vi "FGV Modbus_F.vi"(6 "Aktion":T1) -> (0 "error out":errorcluster)   [LabVIEW 2020, in "ABB-EL3000.lvlib" / "FID.lvlib"]
uses:
  FID.lvlib
  Aktion FGV Modbus_F.ctl
  Aktion Adressen_F.ctl
  Aktion STY_MES.ctl
  Aktion FGV Messwerte_F.ctl
  Allgemeine VI/Aktion Modbus lesen.ctl
  Status Analysatoren/Aktion Status Analysatoren.ctl
  FID Kalibrierung/Aktion FID Allgemeindaten.ctl
  Allgemeine VI/Allgemeine VI.lvlib
  FID Kalibrierung/FID Kalibrierung.lvlib
  Status Analysatoren/Status Analysatoren.lvlib
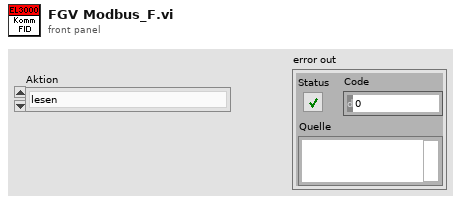
[diagram p1: front panel]
types:
  T1 = typedef "ABB-EL3000.lvlib/FID.lvlib/Aktion FGV Modbus_F.ctl" = enum16{"lesen", "Verbindung herstellen", "Verbindung trennen", "Komm"}
  T2 = typedef "ABB-EL3000.lvlib/FID.lvlib/Aktion Adressen_F.ctl" = enum16{"lesen", "initialisieren"}
  T3 = typedef "Status Analysatoren.lvlib/Aktion Status Analysatoren.ctl" = enum16{"lesen", "initialisieren", "Analysatoren aktiv", "FTIR Fehler", "FID Fehler", "PMA Fehler", "Felder einfärben"}
  T4 = typedef "ABB-EL3000.lvlib/Allgemeine VI.lvlib/Aktion Modbus lesen.ctl" = enum16{"Coils", "Discrete Inputs", "Input Register", "Holding Register"}
  T5 = typedef "ABB-EL3000.lvlib/FID.lvlib/Aktion FGV Messwerte_F.ctl" = enum16{"lesen", "Messwerte", "Messbereich", "Status", "Diagnose Werte"}
  T6 = typedef "Aktion STY_MES.ctl" = enum16{"lesen", "setze STY", "setze MES", "MODBUS schreiben"}
  T7 = typedef "ABB-EL3000.lvlib/FID.lvlib/FID Kalibrierung.lvlib/Aktion FID Allgemeindaten.ctl" = enum16{"lesen", "Mod", "Time", "laden", "speichern"}
  T8 = typedef "Status Analysatoren.lvlib/Status.ctl" = cluster{"FT-IR aktiv":bool, "FT-IR Fehler":bool, "FID aktiv":bool, "FID Fehler":bool, "PMA aktiv":bool, "PMA Fehler":bool}
  T9 = typedef "ABB-EL3000.lvlib/FID.lvlib/Modus.ctl" = enum16{"Automatic", "CH4", "THC", "Efficienty measure", "Switching time"}
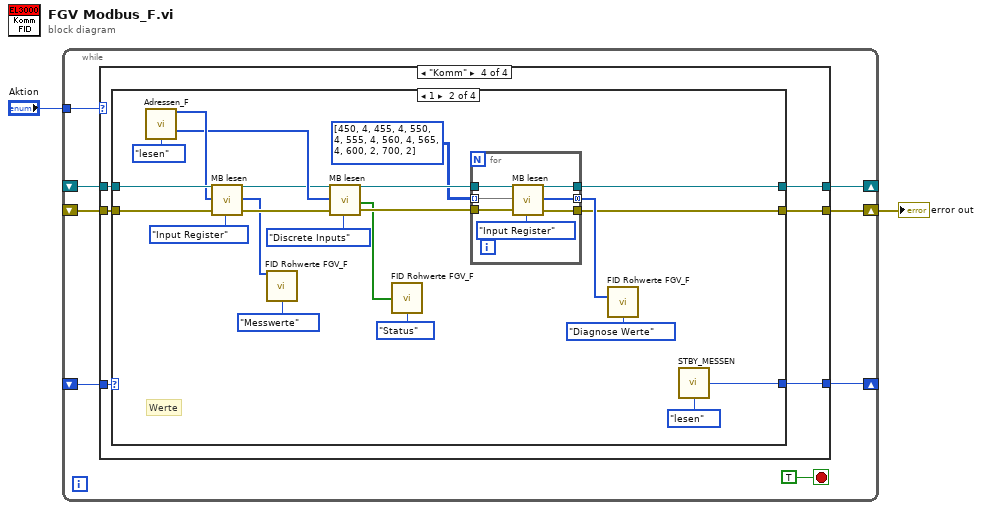
[diagram p0: block diagram]
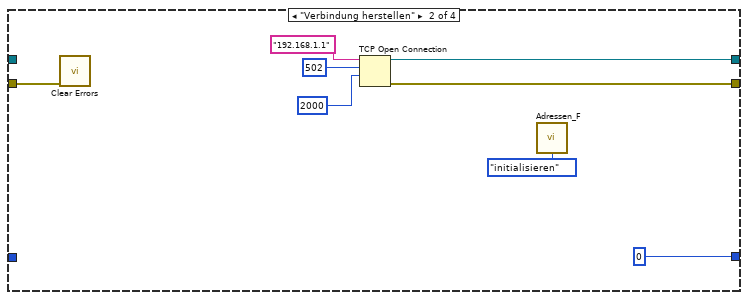
[diagram p3: hidden frame]
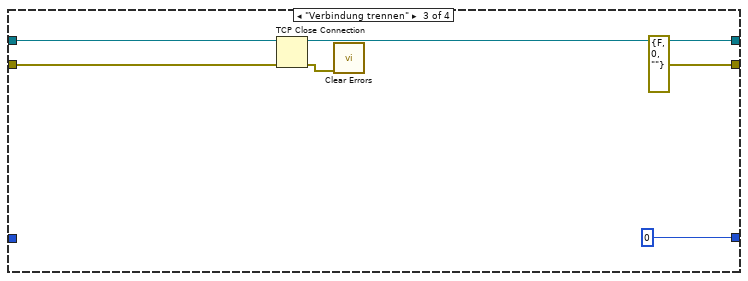
[diagram p4: hidden frame]
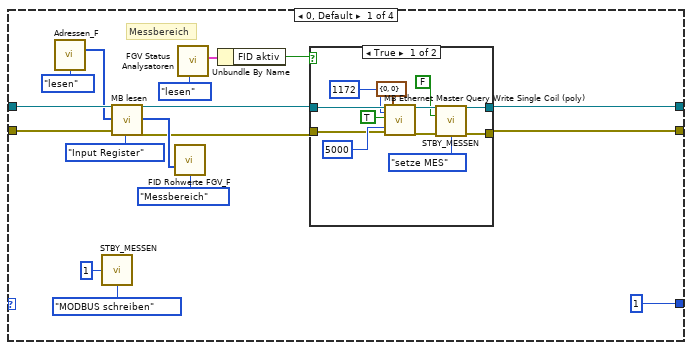
[diagram p5: hidden frame]
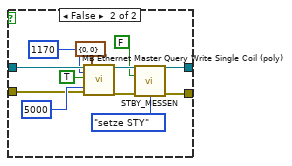
[diagram p6: hidden frame]
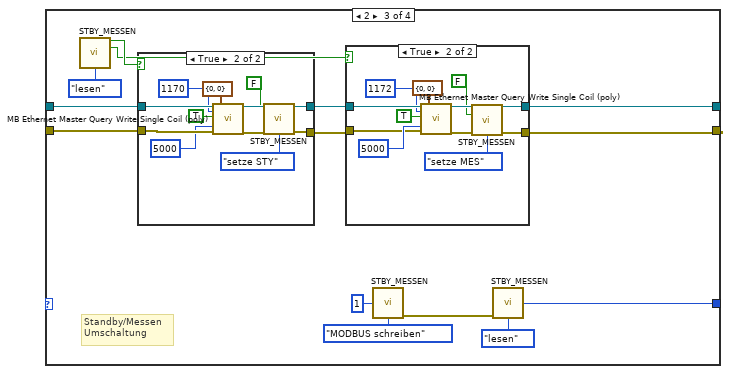
[diagram p7: hidden frame]
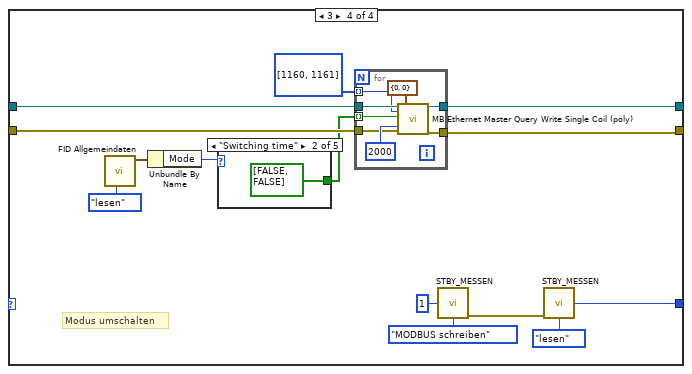
[diagram p10: hidden frame]
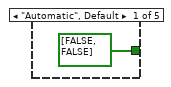
[diagram p11: hidden frame]
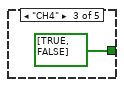
[diagram p12: hidden frame]
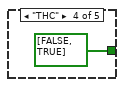
[diagram p13: hidden frame]
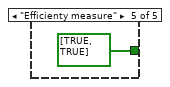
[diagram p14: hidden frame]
diagram:
  n1 = while {
    tunnel: "Aktion" -> [w9]
    shift-right: [w8] -> _
    shift-left: _ -> [w7]
    shift-right: [w6] -> w1
    shift-left: _ -> [w5]
    shift-right: [w3] -> _
    shift-left: _ -> [w4]
    stop <- TRUE stop-if-true
    n2 = case shown="\"Komm\"" w9 {
      tunnel: [w13 w20 w25 w32] -> w8
      tunnel: w7 -> [w13 _ w27 w33]
      tunnel: [w12 w19 errorcluster {"status"=FALSE, "code"=0, "source"=""} ("error out") w30] -> w6
      tunnel: w5 -> [w12 w18 w26 w31]
      tunnel: w4 -> [w11 _ _ w29]
      tunnel: [w11 0 0 w28] -> w3
      frame "lesen", Default {
      }
      frame "Verbindung herstellen" {
        n3 = call <vilib>:"Clear Errors.vi"("error in (no error)"=w18) -> ()  [unwired: 5 in, 2 out]
        n4 = TCP Open Connection(address="192.168.1.1" ("Adresse"), remote port or service name=u16 502 ("Netzwerk-Port oder -Dienst"), timeout ms (60000)=2000 ("Timeout in ms (60000)")) -> (connection ID=w20:refnum<k5>, error out=w19:errorcluster)  [unwired: 2 in]
        n5 = call "Adressen_F.vi"("Aktion"=Aktion_Adressen_F."initialisieren") -> ()  [unwired: 11 in, 4 out]
      }
      frame "Verbindung trennen" {
        n6 = TCP Close Connection(connection ID=w27, error in (no error)=w26) -> (connection ID out=w25:refnum<k5>, error out=w23:errorcluster)  [unwired: 1 in]
        n7 = call <vilib>:"Clear Errors.vi"("error in (no error)"=w23) -> ()  [unwired: 5 in, 2 out]
      }
      frame "Komm" {
        n8 = case shown="1" w29 {
          tunnel: w33 -> [w50 w94 w115 w153]
          tunnel: [w35 w74 w106 w152] -> w32
          tunnel: w31 -> [w49 w93 w114 w151]
          tunnel: [w34 w73 w107 w150] -> w30
          tunnel: [1 w80 w110 w154] -> w28
          frame 0, Default {
            # "Messbereich"
            n9 = call "Adressen_F.vi"("Aktion"=Aktion_Adressen_F."lesen") -> ("Messbereich"=w45:u16[])  [unwired: 11 in, 3 out]
            n10 = call "STBY_MESSEN.vi"("Case Nr."=1, "Aktion"=Aktion_STY_MES."MODBUS schreiben") -> ()  [unwired: 10 in, 4 out]
            n11 = call "MB lesen.vi"("TCP Refnum"=w50, "Adresse"=w45, "error in"=w49, "Aktion"=Aktion_Modbus_lesen."Input Register") -> ("TCP Refnum"=w40:refnum<k5>, "Input Registers"=w46:u16[], "error out"=w39:errorcluster)  [unwired: 17 in, 4 out]
            n12 = call "FID Rohwerte FGV_F.vi"("Messbereich"=w46, "Aktion"=Aktion_FGV_Messwerte_F."Messbereich") -> ()  [unwired: 10 in, 4 out]
            n13 = call "FGV Status Analysatoren.vi"("Aktionen"=Aktion_Status_Analysatoren."lesen") -> ("Status Analysatoren"=w37:T8)  [unwired: 10 in]
            n14 = Unbundle By Name(w37) -> ("FID aktiv"=w36:bool)
            n15 = case shown="True" w36 {
              tunnel: w40 -> [w61 w72]
              tunnel: w39 -> [w53 w64]
              tunnel: [w60 w71] -> w35
              tunnel: [w51 w62] -> w34
              frame True {
                n16 = call <userlib>:"MB Ethernet Master Query Write Single Coil (poly).vi"("TCP Connection Refnum in"=w61, "Address"=u16 1172, "Coil"=TRUE, "Timeout"=u32 5000, "error in"=w53, "MBAP Header"=cluster{"Transaction ID":u16, "Unit ID":u8} {"Transaction ID"=0, "Unit ID"=0}) -> ("TCP Connection Refnum (dup)"=w60:refnum<k5>, "error out"=w55:errorcluster)  [unwired: 11 in, 1 out]
                n17 = call "STBY_MESSEN.vi"("Messen"=FALSE, "error in (no error)"=w55, "Aktion"=Aktion_STY_MES."setze MES") -> ("error out"=w51:errorcluster)  [unwired: 9 in, 3 out]
              }
              frame False {
                n18 = call <userlib>:"MB Ethernet Master Query Write Single Coil (poly).vi"("TCP Connection Refnum in"=w72, "Address"=u16 1170, "Coil"=TRUE, "Timeout"=u32 5000, "error in"=w64, "MBAP Header"=cluster{"Transaction ID":u16, "Unit ID":u8} {"Transaction ID"=0, "Unit ID"=0}) -> ("TCP Connection Refnum (dup)"=w71:refnum<k5>, "error out"=w66:errorcluster)  [unwired: 11 in, 1 out]
                n19 = call "STBY_MESSEN.vi"("Messen"=FALSE, "error in (no error)"=w66, "Aktion"=Aktion_STY_MES."setze STY") -> ("error out"=w62:errorcluster)  [unwired: 9 in, 3 out]
              }
            }
          }
          frame 1 {
            # "Werte"
            n20 = call "Adressen_F.vi"("Aktion"=Aktion_Adressen_F."lesen") -> ("Messwerte"=w91:u16[], "Gerätestatus"=w87:u16[])  [unwired: 11 in, 2 out]
            n21 = call "MB lesen.vi"("TCP Refnum"=w94, "Adresse"=w91, "error in"=w93, "Aktion"=Aktion_Modbus_lesen."Input Register") -> ("TCP Refnum"=w85:refnum<k5>, "Input Registers"=w84:u16[], "error out"=w86:errorcluster)  [unwired: 17 in, 4 out]
            n22 = call "FID Rohwerte FGV_F.vi"("Messwerte"=w84, "Aktion"=Aktion_FGV_Messwerte_F."Messwerte") -> ()  [unwired: 10 in, 4 out]
            n23 = call "MB lesen.vi"("TCP Refnum"=w85, "Adresse"=w87, "error in"=w86, "Aktion"=Aktion_Modbus_lesen."Discrete Inputs") -> ("TCP Refnum"=w90:refnum<k5>, "Discrete Inputs"=w83:bool[], "error out"=w89:errorcluster)  [unwired: 17 in, 4 out]
            n24 = call "FID Rohwerte FGV_F.vi"("Status"=w83, "Aktion"=Aktion_FGV_Messwerte_F."Status") -> ()  [unwired: 10 in, 4 out]
            n25 = for {
              tunnel: w90 -> [w101]
              tunnel: w89 -> [w100]
              tunnel: u16[][] [[450, 4], [455, 4], [550, 4], [555, 4], [560, 4], [565, 4], [600, 2], [700, 2]] ("Adresse") -> [w99] mode=indexing
              tunnel: [w98] -> w74
              tunnel: [w97] -> w73
              tunnel: [w96] -> w82 mode=concatenating
              n26 = call "MB lesen.vi"("TCP Refnum"=w101, "Adresse"=w99, "error in"=w100, "Aktion"=Aktion_Modbus_lesen."Input Register") -> ("TCP Refnum"=w98:refnum<k5>, "Input Registers"=w96:u16[], "error out"=w97:errorcluster)  [unwired: 17 in, 4 out]
            }
            n27 = call "FID Rohwerte FGV_F.vi"("Diagnose Werte"=w82, "Aktion"=Aktion_FGV_Messwerte_F."Diagnose Werte") -> ()  [unwired: 10 in, 4 out]
            n28 = call "STBY_MESSEN.vi"("Aktion"=Aktion_STY_MES."lesen") -> ("Case Nr."=w80:i32)  [unwired: 11 in, 3 out]
          }
          frame 2 {
            # "Standby/Messen\nUmschaltung"
            n29 = call "STBY_MESSEN.vi"("Aktion"=Aktion_STY_MES."lesen") -> ("Standby"=w113:bool, "Messen"=w105:bool)  [unwired: 11 in, 2 out]
            n30 = case shown="True" w113 {
              tunnel: w115 -> [w130 w141]
              tunnel: w114 -> [w129 w140]
              tunnel: [w130 w139] -> w109
              tunnel: [w129 w131] -> w108
              frame False {
              }
              frame True {
                n31 = call <userlib>:"MB Ethernet Master Query Write Single Coil (poly).vi"("TCP Connection Refnum in"=w141, "Address"=u16 1170, "Coil"=TRUE, "Timeout"=u32 5000, "error in"=w140, "MBAP Header"=cluster{"Transaction ID":u16, "Unit ID":u8} {"Transaction ID"=0, "Unit ID"=0}) -> ("TCP Connection Refnum (dup)"=w139:refnum<k5>, "error out"=w134:errorcluster)  [unwired: 11 in, 1 out]
                n32 = call "STBY_MESSEN.vi"("Standby"=FALSE, "error in (no error)"=w134, "Aktion"=Aktion_STY_MES."setze STY") -> ("error out"=w131:errorcluster)  [unwired: 9 in, 3 out]
              }
            }
            n33 = case shown="True" w105 {
              tunnel: w109 -> [w117 w128]
              tunnel: w108 -> [w116 w120]
              tunnel: [w117 w127] -> w106
              tunnel: [w116 w118] -> w107
              frame False {
              }
              frame True {
                n34 = call <userlib>:"MB Ethernet Master Query Write Single Coil (poly).vi"("TCP Connection Refnum in"=w128, "Address"=u16 1172, "Coil"=TRUE, "Timeout"=u32 5000, "error in"=w120, "MBAP Header"=cluster{"Transaction ID":u16, "Unit ID":u8} {"Transaction ID"=0, "Unit ID"=0}) -> ("TCP Connection Refnum (dup)"=w127:refnum<k5>, "error out"=w122:errorcluster)  [unwired: 11 in, 1 out]
                n35 = call "STBY_MESSEN.vi"("Messen"=FALSE, "error in (no error)"=w122, "Aktion"=Aktion_STY_MES."setze MES") -> ("error out"=w118:errorcluster)  [unwired: 9 in, 3 out]
              }
            }
            n36 = call "STBY_MESSEN.vi"("Case Nr."=1, "Aktion"=Aktion_STY_MES."MODBUS schreiben") -> ("error out"=w102:errorcluster)  [unwired: 10 in, 3 out]
            n37 = call "STBY_MESSEN.vi"("error in (no error)"=w102, "Aktion"=Aktion_STY_MES."lesen") -> ("Case Nr."=w110:i32)  [unwired: 10 in, 3 out]
          }
          frame 3 {
            # "Modus umschalten"
            n38 = call "FID Allgemeindaten.vi"("Aktion"=Aktion_FID_Allgemeindaten."lesen") -> ("FID Allgemein"=w147:cluster{"Mode":T9, "Switching time":sgl})  [unwired: 9 in, 1 out]
            n39 = Unbundle By Name(w147) -> ("Mode"=w142:T9)
            n40 = case shown="\"Switching time\"" w142 {
              tunnel: [bool[] [FALSE, FALSE] bool[] [FALSE, FALSE] bool[] [TRUE, FALSE] bool[] [FALSE, TRUE] bool[] [TRUE, TRUE]] -> w146
              frame "Automatic", Default {
              }
              frame "Switching time" {
              }
              frame "CH4" {
              }
              frame "THC" {
              }
              frame "Efficienty measure" {
              }
            }
            n41 = for {
              tunnel: w153 -> [w166]
              tunnel: [w165] -> w152
              tunnel: w151 -> [w164]
              tunnel: [w163] -> w150
              tunnel: u16[] [1160, 1161] -> [w162] mode=indexing
              tunnel: w146 -> [w161] mode=indexing
              n42 = call <userlib>:"MB Ethernet Master Query Write Single Coil (poly).vi"("TCP Connection Refnum in"=w166, "Address"=w162, "Coil"=w161, "Timeout"=u32 2000, "error in"=w164, "MBAP Header"=cluster{"Transaction ID":u16, "Unit ID":u8} {"Transaction ID"=0, "Unit ID"=0}) -> ("TCP Connection Refnum (dup)"=w165:refnum<k5>, "error out"=w163:errorcluster)  [unwired: 11 in, 1 out]
            }
            n43 = call "STBY_MESSEN.vi"("Case Nr."=1, "Aktion"=Aktion_STY_MES."MODBUS schreiben") -> ("error out"=w143:errorcluster)  [unwired: 10 in, 3 out]
            n44 = call "STBY_MESSEN.vi"("error in (no error)"=w143, "Aktion"=Aktion_STY_MES."lesen") -> ("Case Nr."=w154:i32)  [unwired: 10 in, 3 out]
          }
        }
      }
    }
  }
  "error out" <- w1
